vi "Send stack info.vi"(8 "error in (no error)":errorcluster, 11 "Tomo in":refnum<class "Tomo.lvclass">) -> (0 "error out":errorcluster, 3 "Tomo out":refnum<class "Tomo.lvclass">)   [LabVIEW 2012, in "Tomo.lvclass"]
uses:
  Tomo.lvclass
  <vilib>/Distrio/Murmex/Murmex/Murmex.lvclass
  <vilib>/Distrio/Murmex/Murmex/update_cluster.ctl
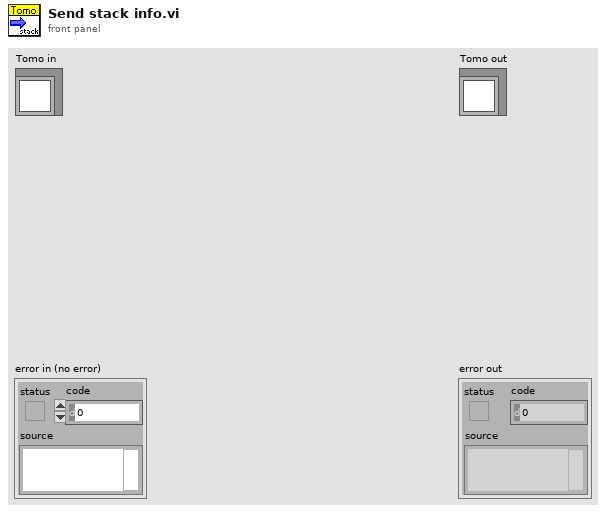
[diagram p1: front panel]
types:
  T1 = typedef "Murmex.lvlib/Murmex.lvclass/update_cluster.ctl" = cluster{"target ID":string, "key chains":string[], "values":variant[]}
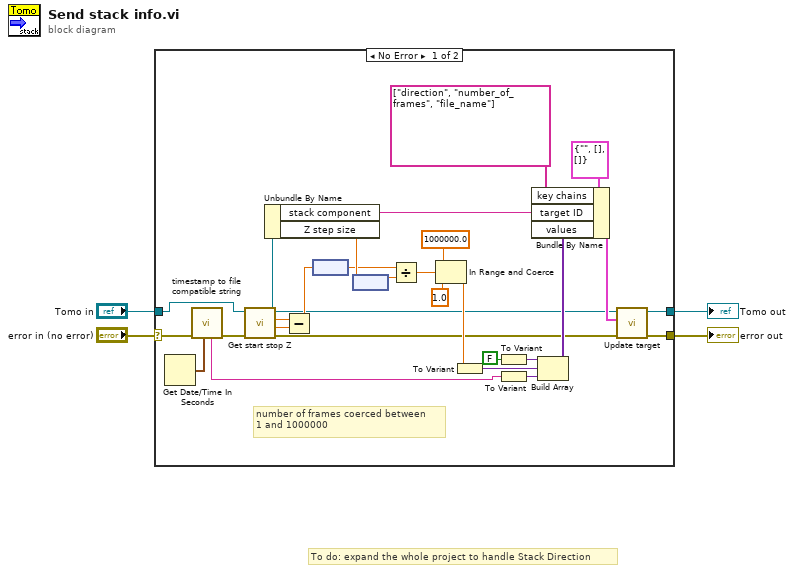
[diagram p0: block diagram]
diagram:
  # "To do: expand the whole project to handle Stack Direction"
  n1 = case shown="No Error" "error in (no error)" {
    selector: "error in (no error)" -> [w8 w34]
    tunnel: [w27 w34] -> w3
    tunnel: [w26 w33] -> w1
    tunnel: "Tomo in" -> [w9 w33]
    frame No Error {
      # "number of frames coerced between\n1 and 1000000"
      n2 = Get Date/Time In Seconds() -> (seconds since 1Jan1904=w6:timestamp)
      n3 = call "timestamp to file compatible string.vi"("time stamp"=w6, "error constant"=w8) -> ("error IO"=w7:errorcluster, "date/time string"=w5:string)  [unwired: 8 in]
      n4 = call-dynamic "Get start stop Z.vi"("error in (no error)"=w7, "Tomo in"=w9) -> ("error out"=w15:errorcluster, "Z start"=w12:dbl[unit], "Z stop"=w13:dbl[unit], "Tomo out"=w14:refnum<class "Tomo.lvclass">)  [unwired: 4 in, 2 out]
      n5 = Unbundle By Name(w14) -> ("stack component"=w24:string, "Z step size"=w32:dbl[unit])
      n6 = Subtract(x=w13, y=w12) -> (x-y=w19:dbl[unit])
      n7 = node(w19) -> (w11:dbl)
      n8 = node(w32) -> (w20:dbl)
      n9 = Divide(x=w11, y=w20) -> (x/y=w10:dbl)
      n10 = In Range and Coerce(upper limit=1000000.0, x=w10, lower limit=1.0) -> (coerced(x)=w18:dbl)  [unwired: 1 out]
      n11 = To Variant(anything=w18) -> (Variant=w30:variant)
      n12 = To Variant(anything=FALSE ("x = 0?")) -> (Variant=w23:variant)
      n13 = To Variant(anything=w5) -> (Variant=w22:variant)
      n14 = Build Array(w23, w30, w22) -> (w29:variant[])
      n15 = Bundle By Name(cluster=T1 {"target ID"="", "key chains"=[], "values"=[]} ("update cluster"), "key chains"=string[] ["direction", "number_of_frames", "file_name"], "target ID"=w24, "values"=w29) -> (w31:T1)
      n16 = call <vilib>:"Update target.vi"("error in (no error)"=w15, "update cluster"=w31, "MurmexBase in"=w14) -> ("error out"=w27:errorcluster, "MurmexBase out"=w26:refnum<class "Tomo.lvclass">)  [unwired: 7 in]
    }
    frame Error {
    }
  }
  "error out" <- w3
  "Tomo out" <- w1
